vi "Condition Tester.vi"() -> ()   [LabVIEW 2016]
uses:
  Support VIs/Draw Water Specific/Type Definitions/HEWH Special Condition Check.ctl
  Type Definitions/PRAT Test.ctl
  Utility/Save File/File Setup (Public)/Type Definition/Save File HEWH Heating Control Mode.ctl
  Support VIs/Draw Water Specific/Type Definitions/Terminate Draw Conditions.ctl
  Type Definitions/HEWH Start Conditions.ctl
  Support VIs/Draw Water Specific/Type Definitions/Check Special Condtions.ctl
  Type Definitions/HEWH Draw Flag ENUM.ctl
  Utility/Save File/File Setup.lvlib
panel:
  in  "index":i32
  in  "Heat-Up Audit Test (50 Gallon)":T1[](array[typedef])=[{"Sequence #"=1.0, "Cycles"=1, "Mode Setting"="Hybrid", "Flow Rate (GPM)"=3.0, "Temperature (F)"=120.0, "Reset Timer"=FALSE, "Use Temp Decline Method"=FALSE, "Terminate Condition"=enum."C1-Terminate Draw @ Gallon Mark", "Condition Value #1"=100.0, "UE"=FALSE, "LE"=FALSE, "Comp"=FALSE, "Fan"=FALSE, "Test End Time (Sec)"=0.0, "Purge Until Cutout"=FALSE, "Start Conditions"=enum."Heat Source Cutout", "Condition Value #2"=0.0, "Remove Power"=FALSE, "Time"=0.0, "Check Special Cond."=enum."SC1-Do Nothing", "Condition#"=enum."N/A", "Draw Flags"=enum."N/A", "Data Processing Delay (FHD 15sec, UEF 5 Sec)"=15.0, "Test Complete"=FALSE}, {"Sequence #"=2.0, "Cycles"=1, "Mode Setting"="Hybrid", "Flow Rate (GPM)"=1.7, "Temperature (F)"=58.0, "Reset Timer"=TRUE, "Use Temp Decline Method"=TRUE, "Terminate Condition"=enum."C1-Terminate Draw @ Gallon Mark", "Condition Value #1"=15.0, "UE"=FALSE, "LE"=FALSE, "Comp"=FALSE, "Fan"=FALSE, "Test End Time (Sec)"=0.0, "Purge Until Cutout"=FALSE, "Start Conditions"=enum."Heat Source Cutout", "Condition Value #2"=0.0, "Remove Power"=FALSE, "Time"=0.0, "Check Special Cond."=enum."SC1-Do Nothing", "Condition#"=enum."N/A", "Draw Flags"=enum."N/A", "Data Processing Delay (FHD 15sec, UEF 5 Sec)"=15.0, "Test Complete"=FALSE}, {"Sequence #"=3.0, "Cycles"=1, "Mode Setting"="Hybrid", "Flow Rate (GPM)"=1.0, "Temperature (F)"=58.0, "Reset Timer"=FALSE, "Use Temp Decline Method"=FALSE, "Terminate Condition"=enum."C1-Terminate Draw @ Gallon Mark", "Condition Value #1"=2.0, "UE"=FALSE, "LE"=FALSE, "Comp"=FALSE, "Fan"=FALSE, "Test End Time (Sec)"=0.0, "Purge Until Cutout"=FALSE, "Start Conditions"=enum."At Time (Seconds)", "Condition Value #2"=1608.0, "Remove Power"=FALSE, "Time"=0.0, "Check Special Cond."=enum."SC1-Do Nothing", "Condition#"=enum."N/A", "Draw Flags"=enum."N/A", "Data Processing Delay (FHD 15sec, UEF 5 Sec)"=15.0, "Test Complete"=FALSE}, {"Sequence #"=4.0, "Cycles"=1, "Mode Setting"="Hybrid", "Flow Rate (GPM)"=1.7, "Temperature (F)"=58.0, "Reset Timer"=FALSE, "Use Temp Decline Method"=FALSE, "Terminate Condition"=enum."C1-Terminate Draw @ Gallon Mark", "Condition Value #1"=9.0, "UE"=FALSE, "LE"=FALSE, "Comp"=FALSE, "Fan"=FALSE, "Test End Time (Sec)"=0.0, "Purge Until Cutout"=FALSE, "Start Conditions"=enum."At Time (Seconds)", "Condition Value #2"=5808.0, "Remove Power"=FALSE, "Time"=0.0, "Check Special Cond."=enum."SC1-Do Nothing", "Condition#"=enum."N/A", "Draw Flags"=enum."N/A", "Data Processing Delay (FHD 15sec, UEF 5 Sec)"=15.0, "Test Complete"=FALSE}, {"Sequence #"=5.0, "Cycles"=1, "Mode Setting"="", "Flow Rate (GPM)"=3.0, "Temperature (F)"=58.0, "Reset Timer"=FALSE, "Use Temp Decline Method"=FALSE, "Terminate Condition"=enum."C9-Do Nothing", "Condition Value #1"=0.0, "UE"=FALSE, "LE"=FALSE, "Comp"=FALSE, "Fan"=FALSE, "Test End Time (Sec)"=0.0, "Purge Until Cutout"=FALSE, "Start Conditions"=enum."Every X (Seconds)", "Condition Value #2"=20.0, "Remove Power"=FALSE, "Time"=0.0, "Check Special Cond."=enum."SC2-Check Heat Source (On-C2/Off-C1)", "Condition#"=enum."N/A", "Draw Flags"=enum."N/A", "Data Processing Delay (FHD 15sec, UEF 5 Sec)"=15.0, "Test Complete"=FALSE}, {"Sequence #"=6.0, "Cycles"=1, "Mode Setting"="", "Flow Rate (GPM)"=3.0, "Temperature (F)"=58.0, "Reset Timer"=FALSE, "Use Temp Decline Method"=FALSE, "Terminate Condition"=enum."C9-Do Nothing", "Condition Value #1"=0.0, "UE"=FALSE, "LE"=FALSE, "Comp"=FALSE, "Fan"=FALSE, "Test End Time (Sec)"=0.0, "Purge Until Cutout"=FALSE, "Start Conditions"=enum."Every X (Seconds)", "Condition Value #2"=600.0, "Remove Power"=FALSE, "Time"=0.0, "Check Special Cond."=enum."SC4-Check Heat Source ON/Fail", "Condition#"=enum."C1", "Draw Flags"=enum."N/A", "Data Processing Delay (FHD 15sec, UEF 5 Sec)"=15.0, "Test Complete"=FALSE}, {"Sequence #"=7.0, "Cycles"=1, "Mode Setting"="", "Flow Rate (GPM)"=3.0, "Temperature (F)"=58.0, "Reset Timer"=FALSE, "Use Temp Decline Method"=FALSE, "Terminate Condition"=enum."C9-Do Nothing", "Condition Value #1"=0.0, "UE"=FALSE, "LE"=FALSE, "Comp"=FALSE, "Fan"=FALSE, "Test End Time (Sec)"=0.0, "Purge Until Cutout"=FALSE, "Start Conditions"=enum."Heat Source Cutout", "Condition Value #2"=0.0, "Remove Power"=FALSE, "Time"=0.0, "Check Special Cond."=enum."SC3-Check Skip Condition", "Condition#"=enum."C1", "Draw Flags"=enum."N/A", "Data Processing Delay (FHD 15sec, UEF 5 Sec)"=15.0, "Test Complete"=FALSE}, {"Sequence #"=8.0, "Cycles"=1, "Mode Setting"="", "Flow Rate (GPM)"=3.0, "Temperature (F)"=58.0, "Reset Timer"=FALSE, "Use Temp Decline Method"=FALSE, "Terminate Condition"=enum."C8-Specific Heat Source", "Condition Value #1"=0.0, "UE"=TRUE, "LE"=FALSE, "Comp"=FALSE, "Fan"=FALSE, "Test End Time (Sec)"=0.0, "Purge Until Cutout"=FALSE, "Start Conditions"=enum."Every X (Seconds)", "Condition Value #2"=600.0, "Remove Power"=FALSE, "Time"=0.0, "Check Special Cond."=enum."SC3-Check Skip Condition", "Condition#"=enum."C1", "Draw Flags"=enum."SmlMedLrg(7)", "Data Processing Delay (FHD 15sec, UEF 5 Sec)"=15.0, "Test Complete"=FALSE}, {"Sequence #"=9.0, "Cycles"=1, "Mode Setting"="", "Flow Rate (GPM)"=3.0, "Temperature (F)"=58.0, "Reset Timer"=FALSE, "Use Temp Decline Method"=FALSE, "Terminate Condition"=enum."C8-Specific Heat Source", "Condition Value #1"=0.0, "UE"=TRUE, "LE"=FALSE, "Comp"=FALSE, "Fan"=FALSE, "Test End Time (Sec)"=0.0, "Purge Until Cutout"=FALSE, "Start Conditions"=enum."Every X (Seconds)", "Condition Value #2"=5.0, "Remove Power"=FALSE, "Time"=0.0, "Check Special Cond."=enum."SC3-Check Skip Condition", "Condition#"=enum."C2", "Draw Flags"=enum."SmlMedLrg(7)", "Data Processing Delay (FHD 15sec, UEF 5 Sec)"=15.0, "Test Complete"=FALSE}, {"Sequence #"=10.0, "Cycles"=1, "Mode Setting"="Hybrid", "Flow Rate (GPM)"=3.0, "Temperature (F)"=58.0, "Reset Timer"=FALSE, "Use Temp Decline Method"=FALSE, "Terminate Condition"=enum."C9-Do Nothing", "Condition Value #1"=0.0, "UE"=FALSE, "LE"=FALSE, "Comp"=FALSE, "Fan"=FALSE, "Test End Time (Sec)"=0.0, "Purge Until Cutout"=FALSE, "Start Conditions"=enum."Wait for UE Cutout", "Condition Value #2"=0.0, "Remove Power"=FALSE, "Time"=0.0, "Check Special Cond."=enum."SC1-Do Nothing", "Condition#"=enum."N/A", "Draw Flags"=enum."N/A", "Data Processing Delay (FHD 15sec, UEF 5 Sec)"=15.0, "Test Complete"=FALSE}, {"Sequence #"=11.0, "Cycles"=1, "Mode Setting"="", "Flow Rate (GPM)"=3.0, "Temperature (F)"=58.0, "Reset Timer"=FALSE, "Use Temp Decline Method"=FALSE, "Terminate Condition"=enum."C9-Do Nothing", "Condition Value #1"=0.0, "UE"=FALSE, "LE"=FALSE, "Comp"=FALSE, "Fan"=FALSE, "Test End Time (Sec)"=0.0, "Purge Until Cutout"=FALSE, "Start Conditions"=enum."Every X (Seconds)", "Condition Value #2"=300.0, "Remove Power"=FALSE, "Time"=0.0, "Check Special Cond."=enum."SC1-Do Nothing", "Condition#"=enum."N/A", "Draw Flags"=enum."N/A", "Data Processing Delay (FHD 15sec, UEF 5 Sec)"=15.0, "Test Complete"=FALSE}, {"Sequence #"=12.0, "Cycles"=1, "Mode Setting"="", "Flow Rate (GPM)"=3.0, "Temperature (F)"=58.0, "Reset Timer"=FALSE, "Use Temp Decline Method"=FALSE, "Terminate Condition"=enum."C9-Do Nothing", "Condition Value #1"=0.0, "UE"=FALSE, "LE"=FALSE, "Comp"=FALSE, "Fan"=FALSE, "Test End Time (Sec)"=0.0, "Purge Until Cutout"=FALSE, "Start Conditions"=enum."Heat Source Cutout", "Condition Value #2"=0.0, "Remove Power"=FALSE, "Time"=0.0, "Check Special Cond."=enum."SC1-Do Nothing", "Condition#"=enum."N/A", "Draw Flags"=enum."N/A", "Data Processing Delay (FHD 15sec, UEF 5 Sec)"=15.0, "Test Complete"=FALSE}, {"Sequence #"=13.0, "Cycles"=1, "Mode Setting"="", "Flow Rate (GPM)"=3.0, "Temperature (F)"=58.0, "Reset Timer"=FALSE, "Use Temp Decline Method"=FALSE, "Terminate Condition"=enum."C9-Do Nothing", "Condition Value #1"=0.0, "UE"=FALSE, "LE"=FALSE, "Comp"=FALSE, "Fan"=FALSE, "Test End Time (Sec)"=0.0, "Purge Until Cutout"=FALSE, "Start Conditions"=enum."Every X (Seconds)", "Condition Value #2"=1800.0, "Remove Power"=FALSE, "Time"=0.0, "Check Special Cond."=enum."SC1-Do Nothing", "Condition#"=enum."N/A", "Draw Flags"=enum."N/A", "Data Processing Delay (FHD 15sec, UEF 5 Sec)"=15.0, "Test Complete"=FALSE}, {"Sequence #"=14.0, "Cycles"=1, "Mode Setting"="", "Flow Rate (GPM)"=3.0, "Temperature (F)"=58.0, "Reset Timer"=FALSE, "Use Temp Decline Method"=FALSE, "Terminate Condition"=enum."C9-Do Nothing", "Condition Value #1"=0.0, "UE"=FALSE, "LE"=FALSE, "Comp"=FALSE, "Fan"=FALSE, "Test End Time (Sec)"=28800.0, "Purge Until Cutout"=FALSE, "Start Conditions"=enum."Heat Source Cutout", "Condition Value #2"=0.0, "Remove Power"=FALSE, "Time"=0.0, "Check Special Cond."=enum."SC1-Do Nothing", "Condition#"=enum."N/A", "Draw Flags"=enum."N/A", "Data Processing Delay (FHD 15sec, UEF 5 Sec)"=15.0, "Test Complete"=FALSE}] {"Time" format="%<%H:%M:%S>t"}
  out "Condition":T6
  out "Trigger Draw Out":bool
  in  "Full Cutout?":bool
  in  "Trigger Draw":bool
  in  "Current Cond":T6
  in  "stop":bool
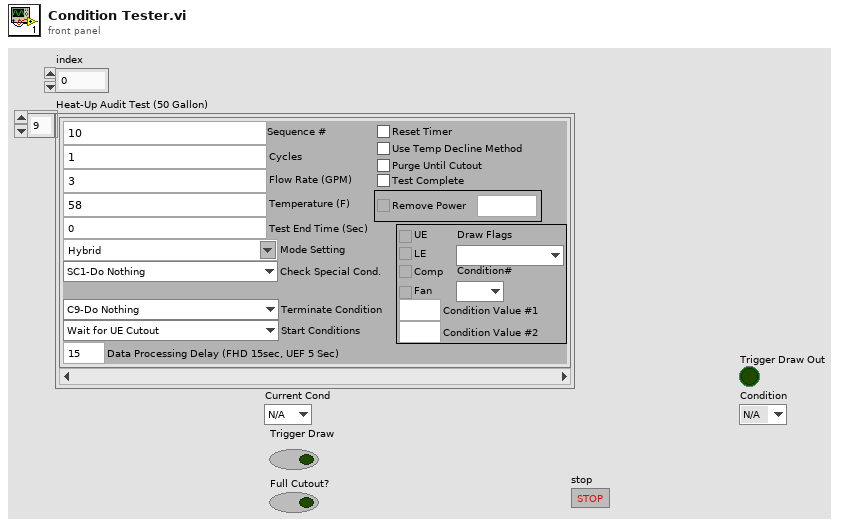
[diagram p1: front panel]
types:
  T1 = typedef "PRAT Test.ctl" = cluster{"Sequence #":dbl, "Cycles":i32, "Mode Setting":T2, "Flow Rate (GPM)":dbl, "Temperature (F)":dbl, "Reset Timer":bool, "Use Temp Decline Method":bool, "Terminate Condition":T3, "Condition Value #1":dbl, "UE":bool, "LE":bool, "Comp":bool, "Fan":bool, "Test End Time (Sec)":dbl, "Purge Until Cutout":bool, "Start Conditions":T4, "Condition Value #2":dbl, "Remove Power":bool, "Time":dbl, "Check Special Cond.":T5, "Condition#":T6, "Draw Flags":T7, "Data Processing Delay (FHD 15sec, UEF 5 Sec)":dbl, "Test Complete":bool}
  T2 = typedef "File Setup.lvlib/Save File HEWH Heating Control Mode.ctl" = string
  T3 = typedef "Terminate Draw Conditions.ctl" = enum16{"C1-Terminate Draw @ Gallon Mark", "C2-Special Last Draw (HU Test)", "C3-RTD Out <=", "C4-Mean Tank Temp <=", "C5-Decrease RTD Out (Deg F)", "C6-Time (Seconds)", "C7-Until Any Heat Source", "C8-Specific Heat Source", "C9-Do Nothing"}
  T4 = typedef "HEWH Start Conditions.ctl" = enum16{"Heat Source Cutout", "At Time (Seconds)", "Every X (Seconds)", "T2 >= X° Below Setpoint", "Seconds From Complete", "Wait for LE & Comp Cutout", "Wait for Comp Cutout", "Wait for LE Cutout", "Wait for UE Cutout"}
  T5 = typedef "Check Special Condtions.ctl" = enum16{"SC1-Do Nothing", "SC2-Check Heat Source (On-C2/Off-C1)", "SC3-Check Skip Condition", "SC4-Check Heat Source ON/Fail"}
  T6 = typedef "HEWH Special Condition Check.ctl" = enum16{"N/A", "C1", "C2", "Reset/Fail", "Skip Draw Sequence"}
  T7 = typedef "HEWH Draw Flag ENUM.ctl" = enum16{"N/A", "None(0)", "Sml(1)", "Med(2)", "SmlMed(3)", "Lrg(4)", "SmlLrg(5)", "MedLrg(6)", "SmlMedLrg(7)"}
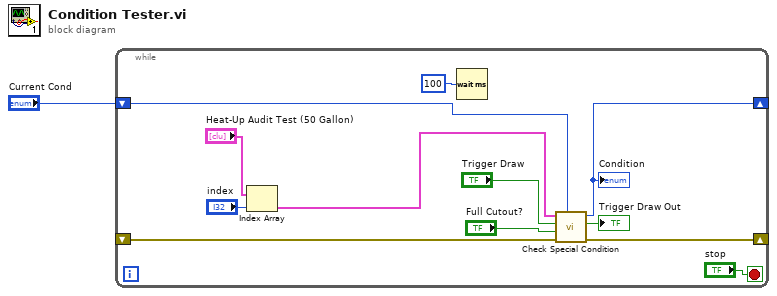
[diagram p0: block diagram]
diagram:
  n1 = while {
    shift-right: [w11] -> _
    shift-left: "Current Cond" -> [w10]
    shift-right: [w6] -> _
    shift-left: _ -> [w7]
    stop <- "stop" stop-if-true
    n2 = Index Array(array="Heat-Up Audit Test (50 Gallon)", index="index") -> (element=w2:T1)
    n3 = Wait (ms)(milliseconds to wait=u32 100) -> ()  [unwired: 1 out]
    n4 = call "Check Special Condition.vi"("Current Cond"=w10, "Error In"=w7, "Full Cutout?"="Full Cutout?", "Trigger Draw"="Trigger Draw", "Station Data Input"=w2) -> ("Error Out"=w6:errorcluster, "Trigger Draw Out"=→"Trigger Draw Out":bool, "Condition"=w11:T6)  [unwired: 4 in]
    "Condition" <- w11
  }
